vi "Load Reference Buffer.vi"(8 "error in (no error)":errorcluster, 9 "Acquired z-plane index":i32, 10 "Ethernet Port Opened ?":bool, 11 "AOL_Globals":T1={"Imaging Protocol"=enum."AOL Z-Stack", "Number of POI"=0, "Number of Miniscans"=0, "Number of Trials"=0, "Number of Cycles "=0, "# Averaged Frames"=0, "Laser power (%)"=0, "Pockels (V)"=0.0, "Acquisition Length (sec)"=0.0, "Fill time (us)"=0.0, "POI Dwell time (us)"=0.0, "Miniscan Dwell time per pixel (us)"=0.0, "PMT 1"=0.0, "PMT 2"=0.0, "Back Apperture (mA)"=200.0, "Frame Size"=0, "Center Frequency"=0.0, "Field of View (um)"=175.0, "Field of View (norm)"=0.0, "DwellTime (us)"=0.0, "Ref Dwell Time (us)"=0.0, "Wavelength (nm)"=0.0, "Zoom"=0.0, "AOL Z"=0.0, "AOL Mode"=enum."Raster", "GridXY"=0.0, "GridZ"=0.0, "TriggerPeriod (sec)"=0.0, "Number of Pixels in Miniscan"=0, "Experiment folder path"=path "", "X centre"=0.0, "Y centre"=0.0, "Angle (degrees)"=0.0, "Angle Xs (degrees)"=0.0, "Angle Ys (degrees)"=0.0, "Plane Mode"=0, "Threshold"=[], "Regenerate Chirps"=FALSE, "Rectangle ROI length (pixels)"=0, "Rectangle ROI height (pixels)"=0, "AOD fill"=4900, "StartupDelay"=0, "Samples Wait after Trigger"=5080, "Slip Cycle"=600000, "Add Cycle"=TRUE, "Functional Mode"=enum."Point", "Z Start"=0.0, "Z Stop"=0.0, "# Planes"=0, "Total Pixels"=0, "Variable Miniscan Pixels"=[], "Use Variable Length"=FALSE, "Use Variable Resolution"=FALSE, "Laser power (%) at Z Start"=0, "Laser power (%) at Z Stop"=0, "Ref Z Step"=0} {"Angle Ys (degrees)" format="%#.6g"; "Angle Xs (degrees)" format="%#.6g"; "Plane Mode" items=["XY Plane", "XZ Plane", "YZ Plane", "arbitraryplane"]; "Frame Size" items=["100X100"=100, "128X128"=128, "200X200"=200, "256X256"=256, "512X512"=512, "1024x1024"=1024, "2048x2048"=2048]; "Back Apperture (mA)" format="%#.6g"; "Pockels (V)" format="%#.6g"; "PMT 2" format="%#.6g"; "PMT 1" format="%#.6g"; "Angle (degrees)" format="%#.6g"; "POI Dwell time (us)" format="%#.6g"}) -> (0 "error out":errorcluster)   [LabVIEW 2020]
uses:
  Typedefs/Controls/AOL_Globals.ctl
  Typedefs/Imaging Protocols enum.ctl
  Typedefs/Frame Size.ctl
  Typedefs/AOL modes.ctl
  Typedefs/Plane Mode.ctl
  Typedefs/Functional Mode.ctl
  Global Variables/General Globals.vi
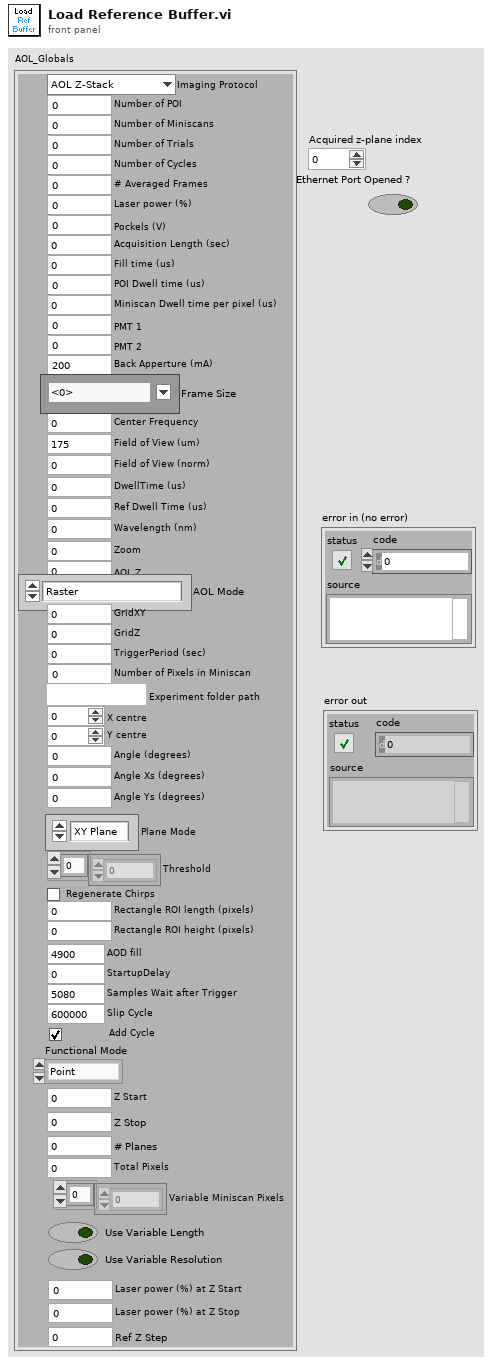
[diagram p1: front panel]
types:
  T1 = typedef "AOL_Globals.ctl" = cluster{"Imaging Protocol":T2, "Number of POI":u16, "Number of Miniscans":u16, "Number of Trials":u16, "Number of Cycles ":u64, "# Averaged Frames":u16, "Laser power (%)":u8, "Pockels (V)":dbl, "Acquisition Length (sec)":dbl, "Fill time (us)":dbl, "POI Dwell time (us)":dbl, "Miniscan Dwell time per pixel (us)":dbl, "PMT 1":dbl, "PMT 2":dbl, "Back Apperture (mA)":dbl, "Frame Size":T3, "Center Frequency":dbl, "Field of View (um)":dbl, "Field of View (norm)":dbl, "DwellTime (us)":dbl, "Ref Dwell Time (us)":dbl, "Wavelength (nm)":dbl, "Zoom":dbl, "AOL Z":dbl, "AOL Mode":T4, "GridXY":dbl, "GridZ":dbl, "TriggerPeriod (sec)":dbl, "Number of Pixels in Miniscan":u16, "Experiment folder path":path, "X centre":dbl, "Y centre":dbl, "Angle (degrees)":dbl, "Angle Xs (degrees)":dbl, "Angle Ys (degrees)":dbl, "Plane Mode":T5, "Threshold":u16[], "Regenerate Chirps":bool, "Rectangle ROI length (pixels)":u16, "Rectangle ROI height (pixels)":u16, "AOD fill":u16, "StartupDelay":i32, "Samples Wait after Trigger":u16, "Slip Cycle":u32, "Add Cycle":bool, "Functional Mode":T6, "Z Start":dbl, "Z Stop":dbl, "# Planes":i32, "Total Pixels":i32, "Variable Miniscan Pixels":u16[], "Use Variable Length":bool, "Use Variable Resolution":bool, "Laser power (%) at Z Start":u8, "Laser power (%) at Z Stop":u8, "Ref Z Step":i8}
  T2 = typedef "Imaging Protocols enum.ctl" = enum16{"AOL Z-Stack", "Motor Z Stack", "Parameter Sweep", "Functional Acquisition", "Single Plane Acquisition", "Volume Acquisition", "Live Imaging", "Live Plane Imaging", "Live Volume Imaging"}
  T3 = typedef "Frame Size.ctl" = u16
  T4 = typedef "AOL modes.ctl" = enum16{"Raster", "Structural", "Pointing", "Mini Scan", "Alignment"}
  T5 = typedef "Plane Mode.ctl" = u16
  T6 = typedef "Functional Mode.ctl" = enum16{"Point", "Line", "Patch", "Plane", "Volume"}
  T7 = cluster{"XYZ Start":cluster{"X":sgl, "Y":sgl, "Z":sgl}[], "XYZ Stop":cluster{"X":sgl, "Y":sgl, "Z":sgl}[]}
  T8 = cluster{"XYZ Coordinates":cluster{"X":sgl, "Y":sgl, "Z":sgl}[], "XYZ Start":cluster{"X":dbl, "Y":dbl, "Z":dbl}[], "XYZ Stop":cluster{"X":dbl, "Y":dbl, "Z":dbl}[]}
  T9 = typedef "Chirp_ABCD.ctl" = cluster{"M ":dbl, "Tramp":dbl[][], "A":dbl[][], "B":dbl[][], "C":dbl[][], "D":dbl[][], "delta_bz":dbl[][], "delta_a_dz":dbl[][], "d_4app":dbl[][], "timings_offsets":dbl[], "distortion_corr":dbl}
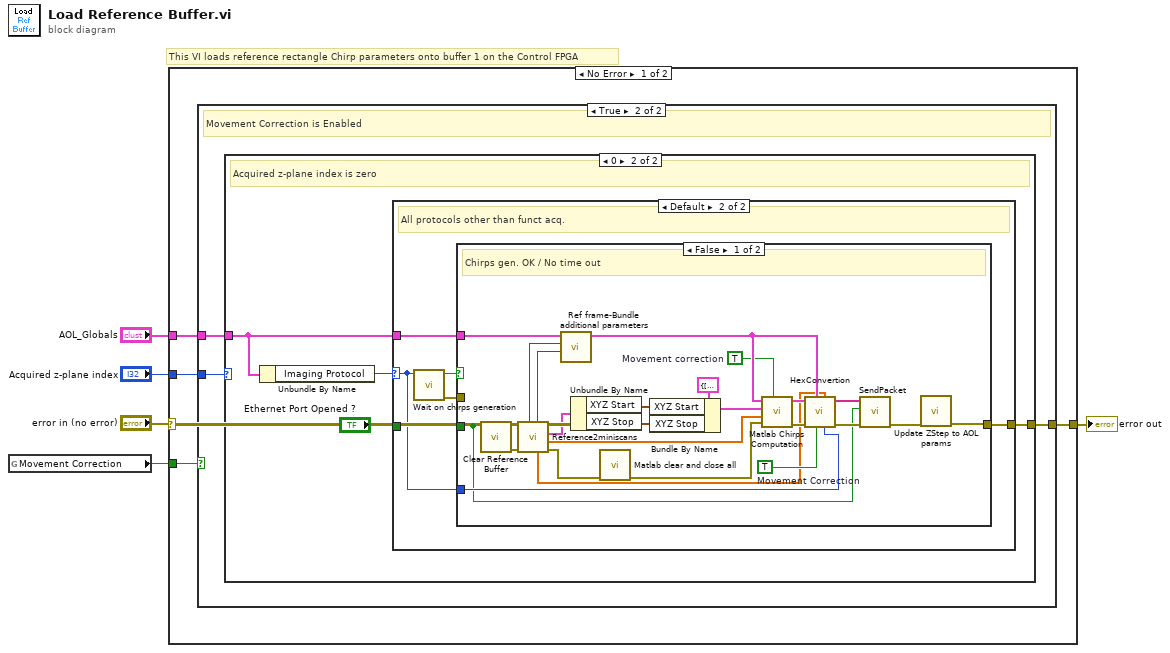
[diagram p0: block diagram]
diagram:
  # "This VI loads reference rectangle Chirp parameters onto buffer 1 on the Control FPGA"
  n1 = global read "General Globals.vi" "Movement Correction"() -> (w1:bool)
  n2 = case shown="No Error" "error in (no error)" {
    selector: "error in (no error)" -> [_ w48]
    tunnel: [w9 w48] -> w4
    tunnel: "AOL_Globals" -> [w8 _]
    tunnel: "Acquired z-plane index" -> [w7 _]
    tunnel: w1 -> [w6 _]
    frame No Error {
      n3 = case shown="True" w6 {
        tunnel: [_ w12] -> w9
        tunnel: w8 -> [_ w11]
        tunnel: w7 -> [_ w10]
        frame False {
          # "Movement Correction is OFF"
        }
        frame True {
          # "Movement Correction is Enabled"
          n4 = case shown="0" w10 {
            tunnel: [_ w16] -> w12
            tunnel: w11 -> [_ w15]
            frame Default {
              # "Acquired z-plane index is anything other than zero"
            }
            frame 0 {
              # "Acquired z-plane index is zero"
              n5 = Unbundle By Name(w15) -> ("Imaging Protocol"=w14:T2)
              n6 = case shown="Default" w14 {
                selector: w14 -> [_ w19]
                tunnel: [_ w22] -> w16
                tunnel: w15 -> [_ w21]
                tunnel: "Ethernet Port Opened ?" -> [_ w17]
                frame "Functional Acquisition" {
                  # "In the functional acquisition case with MC the reference frame's buffer will have already been loaded during AOL Z-stack.\n\nRe-loading the ref buffer here would cause the MC to lose tracking. This has been confirmed by actual testing.\n\nNote that for the buffer to be loaded a Z-stack must be run without MC, then the ref frame must be selected, and then another Z-stack must be run while MC is on to select ROIs."
                }
                frame Default {
                  # "All protocols other than funct acq."
                  n7 = call "Wait on chirps generation.vi"("Imaging Protocol"=w19) -> ("error out"=w18:errorcluster, "Timed out waiting on Chirps generation"=w20:bool)  [unwired: 9 in]
                  n8 = case shown="False" w20 {
                    tunnel: [w23 w47] -> w22
                    tunnel: w21 -> [w46 _]
                    tunnel: w19 -> [w31 _]
                    tunnel: w18 -> [_ w47]
                    tunnel: w17 -> [w26 _]
                    frame False {
                      w25 = TRUE  # Movement correction
                      w28 = TRUE  # Movement Correction
                      # "Chirps gen. OK / No time out"
                      n9 = call "Clear Reference Buffer.vi"("Ethernet port opened"=w26) -> ("error out"=w36:errorcluster)  [unwired: 10 in]
                      n10 = call "Reference2miniscans.vi"("error in (no error)"=w36) -> ("error out"=w30:errorcluster, "Ref Zoom"=w35:dbl[], "miniScan_Coordinates"=w38:T8, "Laser(V)"=w27:dbl[], "No of Miniscans"=w33:i32, "No of Pixels"=w34:i32)  [unwired: 4 in, 1 out]
                      n11 = call "Ref frame-Bundle additional parameters.vi"("No of Miniscans"=w33, "No of Pixels"=w34, "AOL_Globals in"=w46) -> ("AOL_Globals out"=w32:T1)  [unwired: 8 in]
                      n12 = Unbundle By Name(w38) -> ("XYZ Start"=w42:cluster{"X":dbl, "Y":dbl, "Z":dbl}[], "XYZ Stop"=w43:cluster{"X":dbl, "Y":dbl, "Z":dbl}[])
                      n13 = call "Matlab clear and close all.vi"("error in (no error)"=w30) -> ("error out"=w29:errorcluster)  [unwired: 10 in]
                      n14 = Bundle By Name(cluster=T7 {"XYZ Start"=[{"X"=0.0, "Y"=0.0, "Z"=0.0}], "XYZ Stop"=[]} ("ROI Coordinates"), "XYZ Start"=w42, "XYZ Stop"=w43) -> (w40:T7)
                      n15 = call "Matlab Chirps Computation.vi"("Movement correction"=w25, "error in"=w29, "Zoom"=w35, "ROI Coordinates"=w40, "AOL_Globals"=w32) -> ("error out"=w45:errorcluster, "Chirp Parameters"=w44:T9)  [unwired: 3 in, 2 out]
                      n16 = call "HexConvertion.vi"("Imaging Protocol"=w31, "Laser(V)"=w27, "Movement Correction"=w28, "AOL_Globals"=w32, "error in (no error)"=w45, "Chirp Parameters"=w44) -> ("error out"=w37:errorcluster, "HexPackets"=w39:string[])  [unwired: 3 in, 1 out]
                      n17 = call "SendPacket.vi"("error in"=w37, "Ethernet Port Opened ?"=w26, "Packet Array"=w39) -> ("error out"=w24:errorcluster)  [unwired: 7 in, 1 out]
                      n18 = call "Update ZStep to AOL params.vi"("error in (no error)"=w24) -> ("error out"=w23:errorcluster)  [unwired: 10 in]
                    }
                    frame True {
                      # "Timed out waiting on chirp parameters generation."
                    }
                  }
                }
              }
            }
          }
        }
      }
    }
    frame Error {
    }
  }
  "error out" <- w4
